vi "Drive Controller.vi"(8 "error in":errorcluster) -> ()   [LabVIEW 2020]
doc: "This VI executes continuously carrying out the current operation and responding to updates or new operation requests. It will often contain the timing or control code that is difficult to place directly in TeleOp. This VI generally opens all sensors and motors and isolates the rest of the robot code from knowing implementation details of how the operations are carried out."
uses:
  <vilib>/Rock Robotics/WPI/Framework/Completion Status.ctl
  Drive Setpoints.ctl
  Drive Operations.ctl
  <vilib>/Rock Robotics/WPI/SafetyOutput/WPI_SafetyOutputConfigMenu.ctl
  <vilib>/Rock Robotics/WPI/RobotDrive/WPI_RobotDriveOpen2MotorWithExistingMotors.vi
  <vilib>/Rock Robotics/Network Tables/NT Write Variant.vi
panel:
  in  "Interactive Values":T1
  in  "Buttons":cluster{"Execute Cmd":bool, "Abort Cmd":bool}
  out "Command Timing":cluster{"Start Time (ms)":u32, "Iterations":i32}
  out "Status":T3
  out "Setpoints":T4(graph)
  out "Current\nCmd":string
  # "Tip: The graph shows the motor setpoints. It may also be helpful to observe inputs and sensor values.\nYou may also want to display tuning or debugging controls."
  # "Interactive Command: You may fill in the settings for a command\nand schedule it with the Execute button. You can observe and abort\nany command while fine tuning the code for the controller."
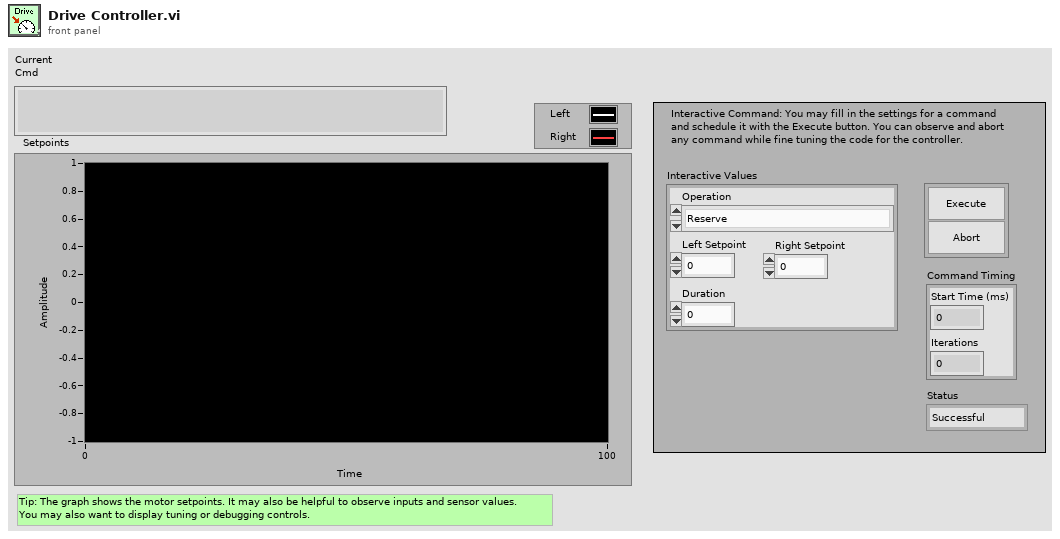
[diagram p1: front panel]
types:
  T1 = typedef "Drive Setpoints.ctl" = cluster{"Operation":T2, "Left Setpoint":dbl, "Right Setpoint":dbl, "Duration":dbl}
  T2 = typedef "Drive Operations.ctl" = enum16{"Reserve", "Read Current", "Immediate", "Drive for Time", "Drive for Distance"}
  T3 = typedef "Completion Status.ctl" = enum16{"Successful", "Aborted", "Incomplete"}
  T4 = cluster{"Left Setpoint":dbl, "Right Setpoint":dbl}
  T5 = typedef "WPI_SafetyOutputConfigMenu.ctl" = enum16{"Enable", "Disable"}
  T6 = typedef "WPI_MotorControlDeviceRef.ctl" = cluster{"DeviceStatus":errorcluster, "Type":T7, "PWM":cluster{"PWM Channel":T8, "DeadBand":T9}, "CAN":cluster{"Device Number":u8, "SetOutput VI Ref":variant, "GetOutput VI Ref":variant, "Enable VI Ref":variant, "Disable VI Ref":variant, "Data":variant}, "Invert":bool, "DIO PWM":cluster{"PWM \"Enable\" Channel":T8, "DIOChannel":T10, "PWM Rate":dbl}}
  T7 = typedef "WPI_MotorControlType.ctl" = enum16{"PWM", "CAN", "DIO PWM"}
  T8 = typedef "FPGA_DIOPWMChannel.ctl" = enum8{"PWM 0", "PWM 1", "PWM 2", "PWM 3", "PWM 4", "PWM 5", "PWM 6", "PWM 7", "PWM 8", "PWM 9", "PWM MXP 0", "PWM MXP 1", "PWM MXP 2", "PWM MXP 3", "PWM MXP 4", "PWM MXP 5", "PWM MXP 6", "PWM MXP 7", "PWM MXP 8", "PWM MXP 9", "Invalid"}
  T9 = typedef "WPI_PWMDeadband.ctl" = cluster{"Name":string, "maxPositivePwm":i32, "minPositivePwm":i32, "centerPwm":i32, "maxNegativePwm":i32, "minNegativePwm":i32, "angularRange":u16}
  T10 = typedef "FPGA_DIOChannel.ctl" = enum8{"DIO 0", "DIO 1", "DIO 2", "DIO 3", "DIO 4", "DIO 5", "DIO 6", "DIO 7", "DIO 8", "DIO 9", "DIO MXP 0", "DIO MXP 1", "DIO MXP 2", "DIO MXP 3", "DIO MXP 4", "DIO MXP 5", "DIO MXP 6", "DIO MXP 7", "DIO MXP 8", "DIO MXP 9", "DIO MXP 10", "DIO MXP 11", "DIO MXP 12", "DIO MXP 13", "DIO MXP 14", "DIO MXP 15", "SPI Port CS1", "SPI Port CS2", "SPI Port CS3", "SPI Port MISO", "SPI Port MOSI", "Invalid"}
  T11 = typedef "WPI_RobotDriveDevRef.ctl" = cluster{"DevStatus":errorcluster, "Motors[]":T6[], "Square Inputs":bool, "Max Output":dbl}
  T12 = typedef "Command Status Info.ctl" = cluster{"Name":string, "Status":T3, "notifier out":T13}
  T13 = typedef "Completion Notifier.ctl" = refnum<notifier>
  T14 = cluster{"SubSystem Data":T1, cluster{"Start Time (ms)":u32, "Iterations":i32}, cluster{"Command Info":T12, "Description":string, "Default Command":T1, "queue out":refnum<queue>, "Subsystem Name":string}}
  T15 = cluster{"SubSystem Data":T1, cluster{"Start Time (ms)":u32, "Iterations":i32}, "Default Command Arguments":cluster{"Command Info":T12, "Description":string, "Default Command":T1, "queue out":refnum<queue>, "Subsystem Name":string}}
  T16 = cluster{"Don't move motors while reserved":dbl, "Don't move motors while reserved":dbl}
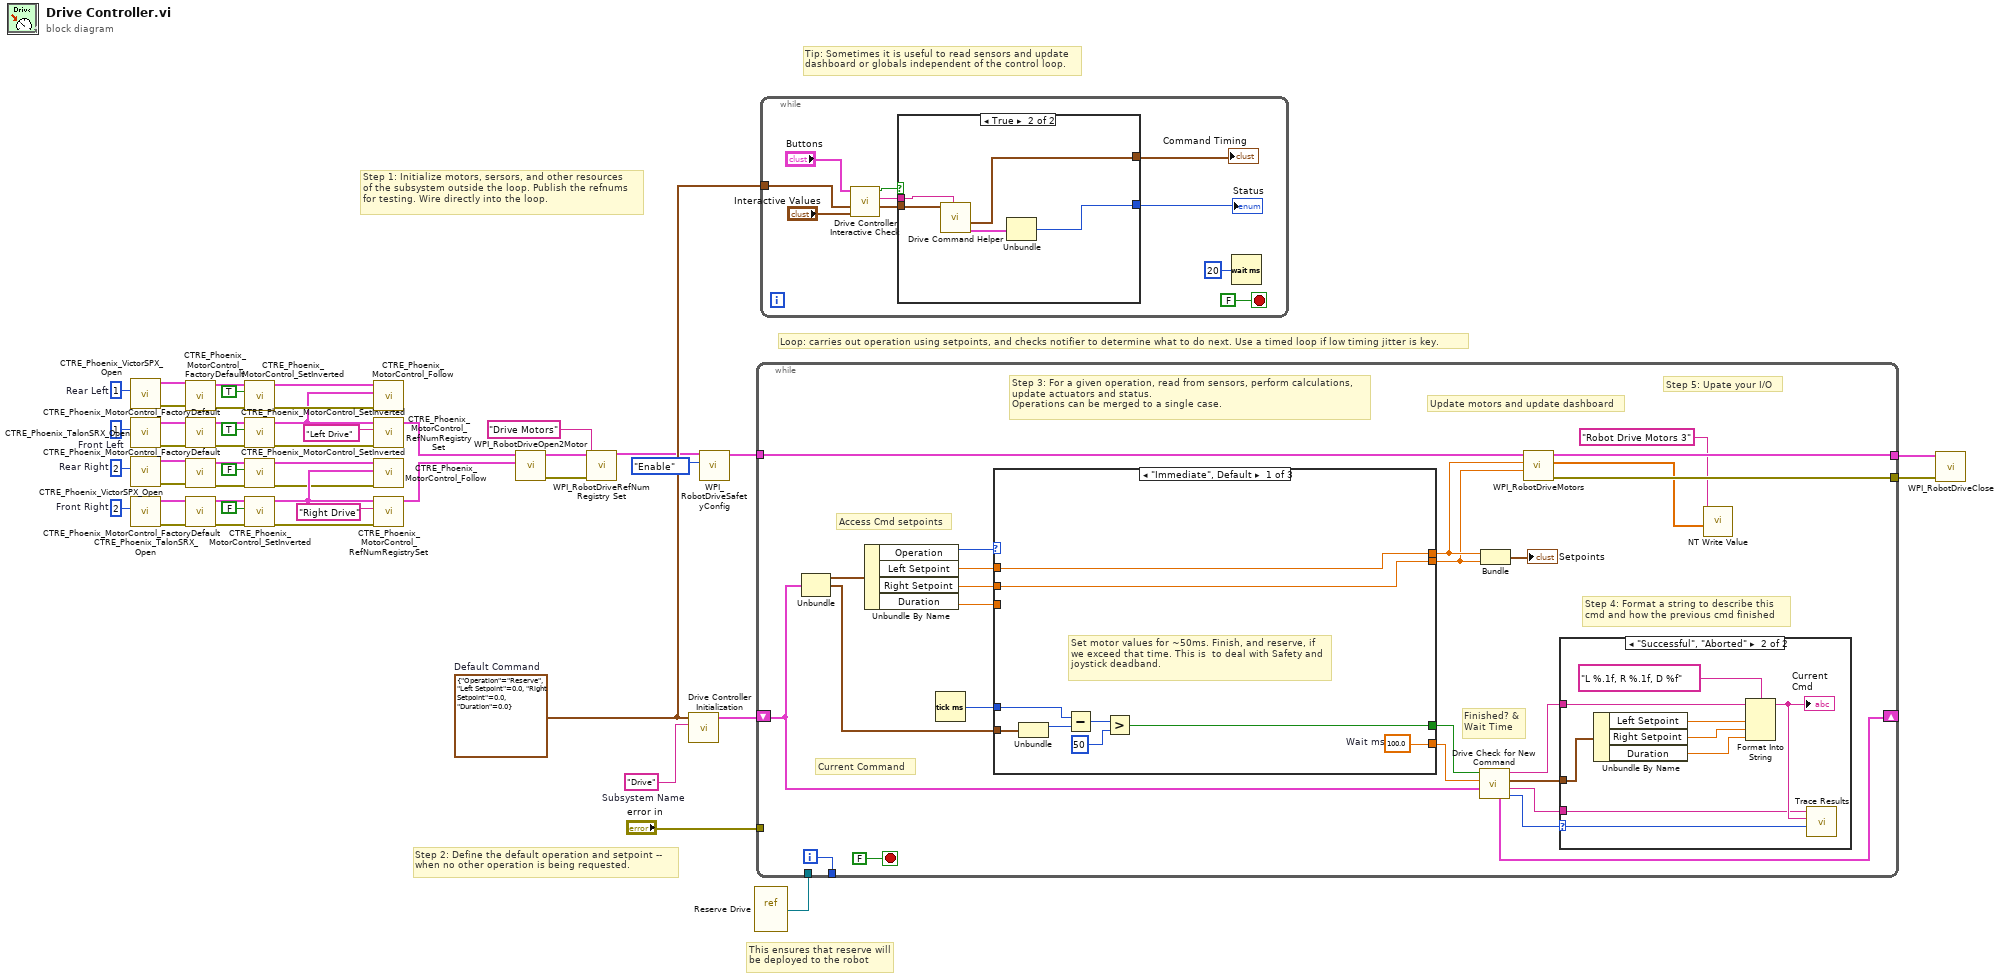
[diagram p0: block diagram]
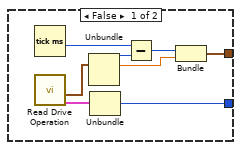
[diagram p2: hidden frame]
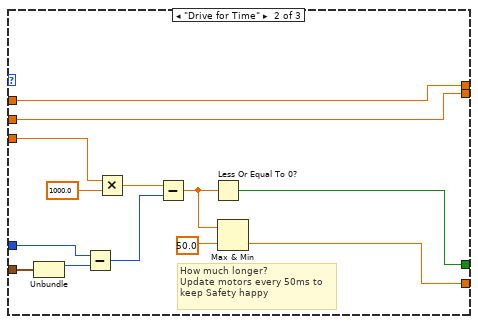
[diagram p4: hidden frame]
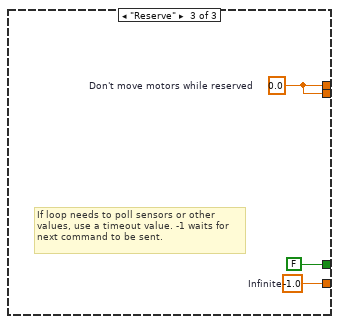
[diagram p5: hidden frame]
diagram:
  w10 = u8 2  # Front Right
  w11 = u8 2  # Rear Right
  w29 = u8 1  # Front Left
  w30 = u8 1  # Rear Left
  w44 = T1 {"Operation"=enum."Reserve", "Left Setpoint"=0.0, "Right Setpoint"=0.0, "Duration"=0.0}  # Default Command
  w49 = "Drive"  # Subsystem Name
  # "This ensures that reserve will\nbe deployed to the robot"
  # "Tip: Sometimes it is useful to read sensors and update\ndashboard or globals independent of the control loop."
  # "Step 2: Define the default operation and setpoint --\nwhen no other operation is being requested."
  # "Step 1: Initialize motors, sersors, and other resources\nof the subsystem outside the loop. Publish the refnums\nfor testing. Wire directly into the loop."
  # "Loop: carries out operation using setpoints, and checks notifier to determine what to do next. Use a timed loop if low timing jitter is key."
  n1 = call <vilib>:"CTRE_Phoenix_VictorSPX_Open.vi"("Device Number"=w30) -> ("error out"=w43:errorcluster, "PhoenixMotorControlDevRef"=w42:T6)  [unwired: 9 in]
  n2 = call <vilib>:"CTRE_Phoenix_TalonSRX_Open.vi"("Device Number"=w29) -> ("error out"=w41:errorcluster, "PhoenixMotorControlDevRef"=w40:T6)  [unwired: 9 in]
  n3 = call <vilib>:"CTRE_Phoenix_VictorSPX_Open.vi"("Device Number"=w11) -> ("error out"=w12:errorcluster, "PhoenixMotorControlDevRef"=w13:T6)  [unwired: 9 in]
  n4 = call <vilib>:"CTRE_Phoenix_TalonSRX_Open.vi"("Device Number"=w10) -> ("error out"=w14:errorcluster, "PhoenixMotorControlDevRef"=w15:T6)  [unwired: 9 in]
  n5 = call <vilib>:"CTRE_Phoenix_MotorControl_FactoryDefault.vi"("error in"=w43, "PhoenixMotorControlDevRef"=w42) -> ("error out"=w39:errorcluster, "PhoenixMotorControlDevRef"=w38:T6)  [unwired: 8 in]
  n6 = call <vilib>:"CTRE_Phoenix_MotorControl_FactoryDefault.vi"("error in"=w41, "PhoenixMotorControlDevRef"=w40) -> ("error out"=w37:errorcluster, "PhoenixMotorControlDevRef"=w36:T6)  [unwired: 8 in]
  n7 = call <vilib>:"CTRE_Phoenix_MotorControl_FactoryDefault.vi"("error in"=w12, "PhoenixMotorControlDevRef"=w13) -> ("error out"=w16:errorcluster, "PhoenixMotorControlDevRef"=w17:T6)  [unwired: 8 in]
  n8 = call <vilib>:"CTRE_Phoenix_MotorControl_FactoryDefault.vi"("error in"=w14, "PhoenixMotorControlDevRef"=w15) -> ("error out"=w18:errorcluster, "PhoenixMotorControlDevRef"=w19:T6)  [unwired: 8 in]
  n9 = call <vilib>:"CTRE_Phoenix_MotorControl_SetInverted.vi"("error in (no error)"=w39, "Invert?"=TRUE, "PhoenixMotorControlDevRef"=w38) -> ("error out"=w35:errorcluster, "PhoenixMotorControlDevRef"=w34:T6)  [unwired: 7 in]
  n10 = call <vilib>:"CTRE_Phoenix_MotorControl_SetInverted.vi"("error in (no error)"=w37, "Invert?"=TRUE, "PhoenixMotorControlDevRef"=w36) -> ("error out"=w33:errorcluster, "PhoenixMotorControlDevRef"=w32:T6)  [unwired: 7 in]
  n11 = call <vilib>:"CTRE_Phoenix_MotorControl_SetInverted.vi"("error in (no error)"=w16, "Invert?"=FALSE, "PhoenixMotorControlDevRef"=w17) -> ("error out"=w20:errorcluster, "PhoenixMotorControlDevRef"=w21:T6)  [unwired: 7 in]
  n12 = call <vilib>:"CTRE_Phoenix_MotorControl_SetInverted.vi"("error in (no error)"=w18, "Invert?"=FALSE, "PhoenixMotorControlDevRef"=w19) -> ("error out"=w22:errorcluster, "PhoenixMotorControlDevRef"=w23:T6)  [unwired: 7 in]
  n13 = call <vilib>:"CTRE_Phoenix_MotorControl_Follow.vi"("error in (no error)"=w35, "Master Controller to Follow"=w32, "PhoenixMotorControlDevRef"=w34) -> ()  [unwired: 7 in, 2 out]
  n14 = call <vilib>:"CTRE_Phoenix_MotorControl_RefNumRegistrySet.vi"("error in (no error)"=w33, "refnum name"="Left Drive", "PhoenixMotorControlDevRef"=w32) -> ("PhoenixMotorControlDevRef"=w4:T6)  [unwired: 7 in, 1 out]
  n15 = call <vilib>:"CTRE_Phoenix_MotorControl_Follow.vi"("error in (no error)"=w20, "Master Controller to Follow"=w23, "PhoenixMotorControlDevRef"=w21) -> ()  [unwired: 7 in, 2 out]
  n16 = call <vilib>:"CTRE_Phoenix_MotorControl_RefNumRegistrySet.vi"("error in (no error)"=w22, "refnum name"="Right Drive", "PhoenixMotorControlDevRef"=w23) -> ("PhoenixMotorControlDevRef"=w3:T6)  [unwired: 7 in, 1 out]
  n17 = call-poly <vilib>:"WPI_RobotDriveOpen2Motor.vi"("Right Motor Dev Ref"=w3, "Left Motor Dev Ref"=w4) -> ("error out"=w7:errorcluster, "RobotDriveDevRef"=w8:T11)  [unwired: 8 in]
  n18 = call <vilib>:"WPI_RobotDriveRefNum Registry Set.vi"("error in (no error)"=w7, "refnum name"="Drive Motors", "RobotDriveDevRef"=w8) -> ("RobotDriveDevRef"=w6:T11)  [unwired: 7 in, 1 out]
  n19 = call "Drive Controller Initialization.vi"("Subsystem Name"=w49, "Default Command"=w44) -> ("Current Command"=w46:T14)  [unwired: 9 in]
  n20 = call <vilib>:"WPI_RobotDriveSafetyConfig.vi"("mode"=WPI_SafetyOutputConfigMenu."Enable", "RobotDriveDevRef"=w6) -> ("RobotDriveDevRef"=w48:T11)  [unwired: 8 in, 1 out]
  n21 = vi-ref "Reserve Drive.vi"() -> (w45:refnum<vi>)
  n22 = while {
    shift-right: [w61] -> _
    shift-left: w46 -> [w54]
    tunnel: [w73] -> _
    tunnel: w48 -> [w69]
    tunnel: "error in" -> [_]
    tunnel: w45 -> [_]
    tunnel: [w53] -> w2
    tunnel: [w52] -> w1
    i -> [w73]
    stop <- FALSE stop-if-true
    # "Step 5: Upate your I/O"
    # "Step 4: Format a string to describe this\ncmd and how the previous cmd finished"
    # "Current Command"
    # "Update motors and update dashboard"
    # "Access Cmd setpoints"
    # "Finished? &\nWait Time"
    # "Step 3: For a given operation, read from sensors, perform calculations,\nupdate actuators and status.\nOperations can be merged to a single case."
    n23 = Unbundle(w54) -> ("SubSystem Data"=w68:T1, w55:cluster{"Start Time (ms)":u32, "Iterations":i32})  [unwired: 1 out]
    n24 = Unbundle By Name(w68) -> ("Operation"=w67:T2, "Left Setpoint"=w66:dbl, "Right Setpoint"=w65:dbl, "Duration"=w64:dbl)
    n25 = Tick Count (ms)() -> (millisecond timer value=w63:u32)
    n26 = case shown="\"Immediate\", Default" w67 {
      tunnel: [w92 w93 w108] -> w60
      tunnel: [w85 w100 FALSE ("ignore previous (F)")] -> w59
      tunnel: w55 -> [w84 w102 _]
      tunnel: [w91 w99 w106] -> w71
      tunnel: [w90 w98 w106] -> w70
      tunnel: w66 -> [w91 w99 _]
      tunnel: w65 -> [w90 w98 _]
      tunnel: w64 -> [_ w97 _]
      tunnel: w63 -> [w86 w96 _]
      frame "Immediate", Default {
        w92 = 100.0  # Wait ms
        # "Set motor values for ~50ms. Finish, and reserve, if\nwe exceed that time. This is  to deal with Safety and\njoystick deadband."
        n27 = Unbundle(w84) -> ("Start Time (ms)"=w87:u32)  [unwired: 1 out]
        n28 = Subtract(x=w86, y=w87) -> (x-y=w88:u32)
        n29 = Greater?(x=w88, y=u8 50 ("Left Motor")) -> (0:w85:bool)
      }
      frame "Drive for Time" {
        # "How much longer?\nUpdate motors every 50ms to\nkeep Safety happy"
        n30 = Unbundle(w102) -> ("Start Time (ms)"=w101:u32)  [unwired: 1 out]
        n31 = Subtract(x=w96, y=w101) -> (x-y=w105:u32)
        n32 = Multiply(x=w97, y=1000.0) -> (x*y=w104:dbl)
        n33 = Subtract(x=w104, y=w105) -> (x-y=w95:dbl)
        n34 = Less Or Equal To 0?(x=w95) -> (x <= 0?=w100:bool)
        n35 = Max & Min(x=w95, y=50.0) -> (min(x,y)=w93:dbl)  [unwired: 1 out]
      }
      frame "Reserve" {
        w106 = 0.0  # Don't move motors while reserved
        w108 = -1.0  # Infinite
        # "If loop needs to poll sensors or other\nvalues, use a timeout value. -1 waits for\nnext command to be sent."
      }
    }
    n36 = call "Drive Check for New Command.vi"("input cluster"=w54, "Wait time (ms)"=w60, "Finished?"=w59) -> ("Completion"=w62:T3, "Subsystem Name"=w56:string, "Current Command"=w57:T1, "Initial Trace String"=w58:string, "Next Command"=w61:T15)  [unwired: 4 in]
    n37 = Bundle("Don't move motors while reserved"=w71, "Don't move motors while reserved"=w70) -> (→"Setpoints":T16)  [unwired: 1 in]
    n38 = call <vilib>:"WPI_RobotDriveMotors.vi"("RightSpeed"=w70, "LeftSpeed"=w71, "RobotDriveDevRef"=w69) -> ("error out"=w52:errorcluster, "Motor Values"=w50:dbl[], "RobotDriveDevRef"=w53:T11)  [unwired: 1 in, 5 out]
    n39 = case shown="\"Successful\", \"Aborted\"" w62 {
      selector: w62 -> [_ w83]
      tunnel: w58 -> [_ w78]
      tunnel: w57 -> [_ w79]
      tunnel: w56 -> [_ w75]
      frame "Incomplete", Default {
        # "Continuing current command"
      }
      frame "Successful", "Aborted" {
        # "Report and setup for next command"
        n40 = Unbundle By Name(w79) -> ("Left Setpoint"=w81:dbl, "Right Setpoint"=w82:dbl, "Duration"=w76:dbl)
        n41 = Format Into String(format string="L %.1f, R %.1f, D %f", initial string=w78, w81, w82, w76) -> (resulting string=w77:string)  [unwired: 1 in, 1 out]
        "Current\nCmd" <- w77
        n42 = call <vilib>:"Trace Results.vi"("Status of previous command"=w83, "Description"=w77, "Subsystem"=w75) -> ()  [unwired: 9 in]
      }
    }
    n43 = call-poly <vilib>:"NT Write Value.vi"("Variant"=w50, "Name"="Robot Drive Motors 3") -> ()  [unwired: 9 in, 1 out]
  }
  n44 = while {
    tunnel: w44 -> [w110]
    stop <- FALSE stop-if-true
    n45 = call "Drive Controller Interactive Check.vi"("Interactive Command In"="Interactive Values", "Default Command"=w110, "Buttons"="Buttons") -> ("Interactive Command Out"=w112:T1, "Trace String"=w113:string, "Schedule"=w114:bool)  [unwired: 6 in]
    n46 = case shown="True" w114 {
      tunnel: [w123 w131] -> w115
      tunnel: [w122 w127] -> w116
      tunnel: w113 -> [_ w129]
      tunnel: w112 -> [_ w128]
      frame False {
        n47 = Tick Count (ms)() -> (millisecond timer value=w126:u32)
        n48 = call "Read Drive Operation.vi"() -> ("Command Info"=w120:T12, "SubSystem Data"=w119:T1)  [unwired: 9 in, 1 out]
        n49 = Unbundle(w119) -> ("Operation"=w124:T2, "Left Setpoint"=w121:dbl)  [unwired: 2 out]
        n50 = Unbundle(w120) -> ("Status"=w123:T3)  [unwired: 2 out]
        n51 = Subtract(x=w126, y=w124) -> (x-y=w125:u32)
        n52 = Bundle(w125, "Left Setpoint"=w121) -> (w122:cluster{u32, "Left Setpoint":dbl})  [unwired: 1 in]
      }
      frame True {
        n53 = call "Drive Command Helper.vi"("Description"=w129, "SubSystem Data"=w128) -> ("Command Info Out"=w130:T12, "Command Timing"=w127:cluster{"Start Time (ms)":u32, "Iterations":i32})  [unwired: 7 in, 1 out]
        n54 = Unbundle(w130) -> ("Status"=w131:T3)  [unwired: 2 out]
      }
    }
    "Status" <- w115
    "Command Timing" <- w116
    n55 = Wait (ms)(milliseconds to wait=u32 20) -> ()  [unwired: 1 out]
  }
  n56 = call <vilib>:"WPI_RobotDriveClose.vi"("error in (no error)"=w1, "RobotDriveDevRef"=w2) -> ()  [unwired: 9 in, 1 out]
